vi "Read Attributes.vi"(11 "UI Panel Launched Msg":refnum<class "UI Panel Launched Msg.lvclass">) -> (2 "Payload":cluster{"VI Refnum":refnum<vi>, "Name":string})   [LabVIEW 2015, in "Chat Window UI Controller.lvlib" / "UI Panel Launched Msg.lvclass"]
uses:
  UI Panel Launched Msg.lvclass
  UI Panel Launched Msg.lvclass/UI Panel Launched Msg.ctl
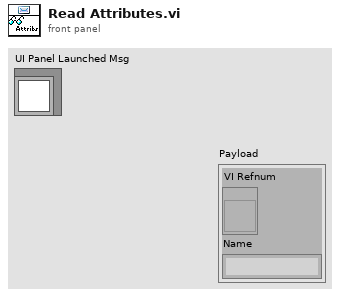
[diagram p1: front panel]
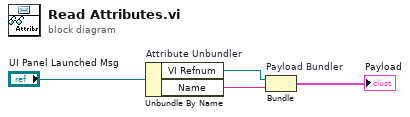
[diagram p0: block diagram]
diagram:
  n1 = Unbundle By Name "Attribute Unbundler"("UI Panel Launched Msg") -> ("VI Refnum"=w2:refnum<vi>, "Name"=w1:string)
  n2 = Bundle "Payload Bundler"("VI Refnum"=w2, "Name"=w1) -> (→"Payload":cluster{"VI Refnum":refnum<vi>, "Name":string})  [unwired: 1 in]
